vi "TestMain.vi"   [LabVIEW 2020]
uses:
  Login-Options.ctl
  Login-UI.lvlib
types:
  T1 = typedef "Login-UI.lvlib/Login-Options.ctl" = cluster{"HideMain(T)":bool, "RetryAllowed(T)":bool, "LastUserToINI(T)":bool, "Titlebar(T)":bool}
  T2 = typedef "Login-UI.lvlib/User-Info.ctl" = cluster{"UserName":string, "Password":string, "Role":T3}
  T3 = typedef "Login-UI.lvlib/User-Role.ctl" = enum16{"INVALID", "Operator", "Engineer", "Admin", "Anonymous"}
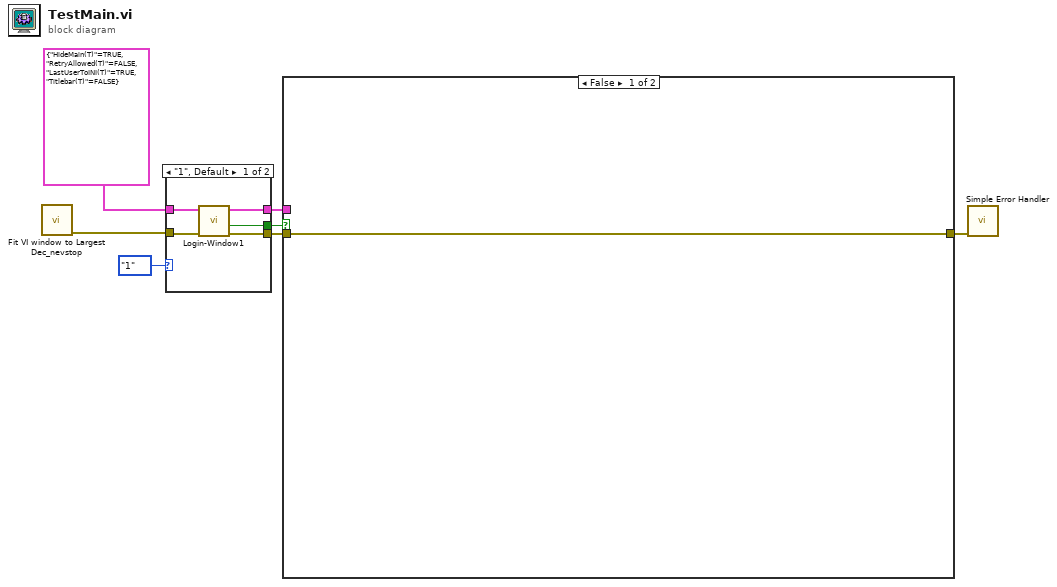
[diagram p0: block diagram]
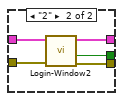
[diagram p2: hidden frame]
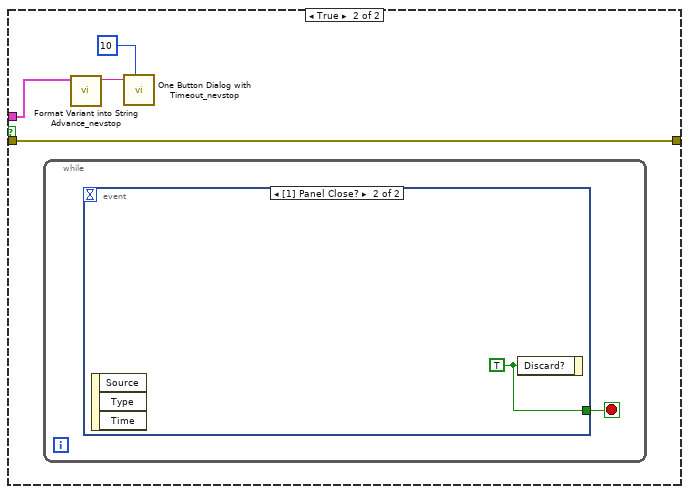
[diagram p3: hidden frame]
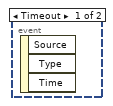
[diagram p4: hidden frame]
diagram:
  n1 = call <userlib>:"Fit VI window to Largest Dec_nevstop.vi"() -> ("error out"=w3:errorcluster)  [unwired: 6 in, 1 out]
  n2 = case shown="\"1\", Default" enum16{"1", "2"}."1" {
    tunnel: [w11 w17] -> w7
    tunnel: [w12 w16] -> w6
    tunnel: [w10 w15] -> w5
    tunnel: w3 -> [w9 w14]
    tunnel: T1 {"HideMain(T)"=TRUE, "RetryAllowed(T)"=FALSE, "LastUserToINI(T)"=TRUE, "Titlebar(T)"=FALSE} ("Options") -> [w8 w13]
    frame "1", Default {
      n3 = call "Login-Window1.vi"("Error in"=w9, "Options"=w8) -> ("Error out"=w10:errorcluster, "Valid User"=w11:bool, "User Info"=w12:T2)  [unwired: 7 in]
    }
    frame "2" {
      n4 = call "Login-Window2.vi"("Error in"=w14, "Options"=w13) -> ("Error out"=w15:errorcluster, "Valid User"=w17:bool, "User Info"=w16:T2)  [unwired: 7 in]
    }
  }
  n5 = case shown="False" w7 {
    tunnel: w6 -> [_ w22]
    tunnel: w5 -> [w18 w19]
    tunnel: [w18 w19] -> w4
    frame False {
    }
    frame True {
      n6 = while {
        stop <- w23 stop-if-true
        n7 = event shown="[1] Panel Close?" {
          selector: _ -> [_ _]
          dyn-events: _ -> [_ _]
          timeout: _ -> [_ _]
          tunnel: [_ w24] -> w23
          event Timeout {
            n8 = event-data() -> ()  [unwired: 1 in, 3 out]
          }
          event Panel Close? {
            w24 = TRUE ("Discard?")
            n9 = event-data() -> ()  [unwired: 1 in, 3 out]
            n10 = event-data("Discard?"=w24) -> ()  [unwired: 1 in, 1 out]
          }
        }
      }
      n11 = call <userlib>:"Format Variant into String Advance_nevstop.vi"("Variant"=w22) -> ("Data"=w21:string)  [unwired: 8 in, 2 out]
      n12 = call <userlib>:"One Button Dialog with Timeout_nevstop.vi"("message"=w21, "Btn Timeout(-1 s)"=10) -> ()  [unwired: 7 in, 1 out]
    }
  }
  n13 = call <vilib>:"Simple Error Handler.vi"("error in (no error)"=w4) -> ()  [unwired: 4 in, 5 out]
